vi "Write Display Format Visible.vi"(5 "Display Format Visible":bool, 9 "String in":refnum<class "String.lvclass">) -> (3 "String out":refnum<class "String.lvclass">)   [LabVIEW 2014, in "Raspberry Pi Compatible Compiler for LabVIEW.lvlib" / "String.lvclass"]
uses:
  String.lvclass
  String.lvclass/String.ctl
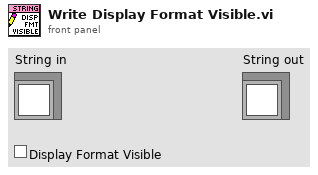
[diagram p1: front panel]
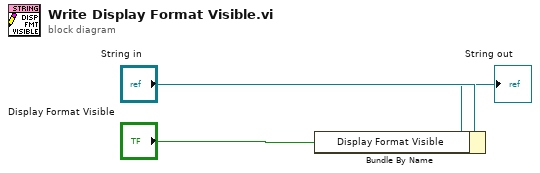
[diagram p0: block diagram]
diagram:
  n1 = Bundle By Name(cluster="String in", "Display Format Visible"="Display Format Visible") -> (→"String out":refnum<class "String.lvclass">)
